vi "disableUnusedSubPanels.vi"(8 "error in (no error)":errorcluster, 11 "Array":refnum<vi>[](array[refnum])) -> ()   [LabVIEW 2013]
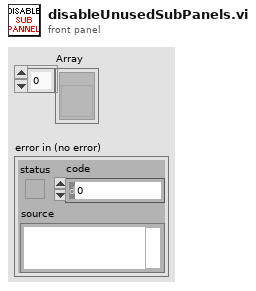
[diagram p1: front panel]
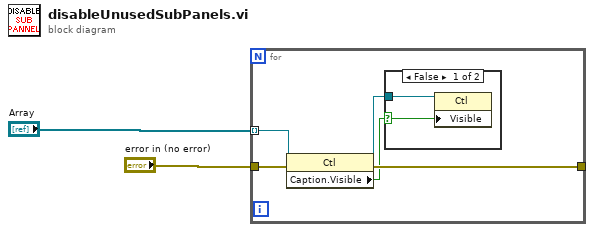
[diagram p0: block diagram]
diagram:
  n1 = for {
    tunnel: "Array" -> [w7] mode=indexing
    tunnel: [w6] -> _
    tunnel: "error in (no error)" -> [w5]
    n2 = property class="Ctl"(reference=w7, error in=w5) -> (reference out=w4:refnum<vi>, error out=w6:errorcluster, "Caption.Visible"=w3:bool)
    n3 = case shown="False" w3 {
      selector: w3 -> [w8 _]
      tunnel: w4 -> [w9 _]
      frame False {
        n4 = property class="Ctl"(reference=w9, "Visible"=w8) -> ()  [unwired: 1 in, 2 out]
      }
      frame True {
      }
    }
  }
